vi "题目7.vi"() -> ()   [LabVIEW 2017]
uses:
  <vilib>/Utility/file.llb/Read Delimited Spreadsheet (DBL).vi
  <vilib>/Analysis/NI_AALBase.lvlib
panel:
  out "all rows":dbl[][](array[numeric]) caption="所有行"
  out "波形图":dbl[](graph)
  out "拆分的路径":path
  in  "cycles":dbl=1.0 caption="周期" format="%0.2f"
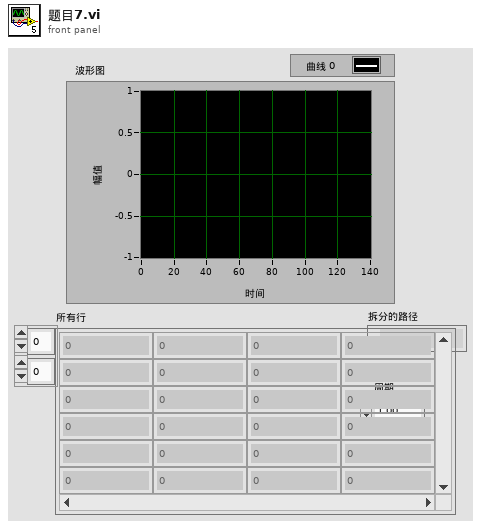
[diagram p1: front panel]
types:
  T1 = enum16{"open", "replace", "create", "open or create", "replace or create", "replace or create with confirmation"}
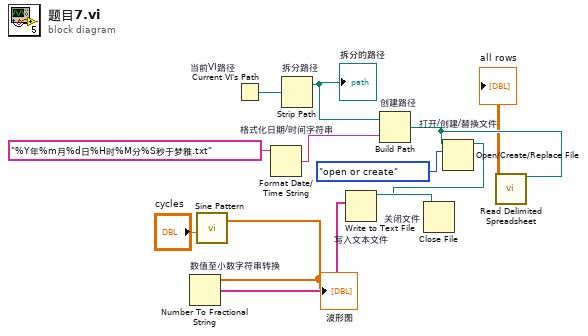
[diagram p0: block diagram]
diagram:
  n1 = call <vilib>:"Sine Pattern.vi"("cycles"="cycles") -> ("Sinusoidal Pattern"=w2:dbl[])  [unwired: 3 in, 1 out]
  "波形图" <- w2
  n2 = Number To Fractional String "数值至小数字符串转换"(number=w2) -> (F-format string=w11:string[])  [unwired: 3 in]
  n3 = Current VI's Path "当前VI路径"() -> (path=w4:path)
  n4 = Format Date/Time String "格式化日期/时间字符串"(time format string (%c)="%Y年%m月%d日%H时%M分%S秒于梦雅.txt" ("时间格式字符串(%c)")) -> (date/time string=w7:string)  [unwired: 2 in]
  n5 = Strip Path "拆分路径"(path=w4) -> (stripped path=w5:path)  [unwired: 1 out]
  "拆分的路径" <- w5
  n6 = Build Path "创建路径"(base path=w5, name or relative path=w7) -> (appended path=w3:path)
  n7 = Open/Create/Replace File "打开/创建/替换文件"(file path (use dialog)=w3, operation (0:open)=T1."open or create" ("操作(0:open)")) -> (refnum out=w9:refnum<file>)  [unwired: 4 in, 2 out]
  n8 = Write to Text File "写入文本文件"(file (use dialog)=w9, text=w11) -> (refnum out=w10:refnum<file>)  [unwired: 2 in, 2 out]
  n9 = Close File "关闭文件"(refnum=w10) -> ()  [unwired: 1 in, 2 out]
  n10 = call-poly <vilib>:"Read Delimited Spreadsheet.vi"("file path (dialog if empty)"=w3) -> ("all rows"=→"all rows":dbl[][])  [unwired: 9 in, 5 out]
